vi "Session Queue FG.vi"(11 "Session Queue In":refnum<queue>) -> (2 "Session Valid?":bool, 3 "Session Queue":refnum<queue>)   [LabVIEW 2020, in "TSnax.lvlib" / "Engine.lvclass"]
uses:
  Engine.lvclass
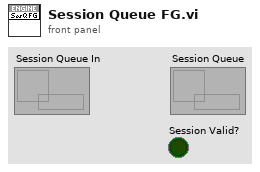
[diagram p1: front panel]
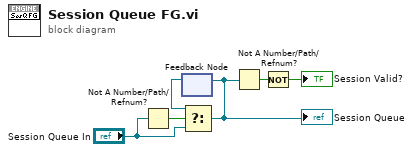
[diagram p0: block diagram]
diagram:
  n1 = Not A Number/Path/Refnum?(number/path/refnum="Session Queue In") -> (NaN/Path/Refnum?=w6:bool)
  n2 = feedback #1() -> (w4:refnum<queue>)  [unwired: 1 in]
  n3 = Select(t=w4, s=w6, f="Session Queue In") -> (s? t:f=w3:refnum<queue>)
  "Session Queue" <- w3
  n4 = feedback-in #1(w3) -> ()
  n5 = Not A Number/Path/Refnum?(number/path/refnum=w3) -> (NaN/Path/Refnum?=w2:bool)
  n6 = Not(x=w2) -> (.not. x?=→"Session Valid?":bool)
